vi "trainer on read.vi"(11 "error in (no error)":errorcluster) -> (8 "Trainer is on":bool, 15 "error out":errorcluster)   [LabVIEW 2016]
doc: "this vi reads the trainer 5V power rail using channel 3 to check that the power is on\n\nPaul K Dixon\nPhysics 350\nPaul K Dixon"
panel:
  in  "channel":tag="Dev1/ai3"
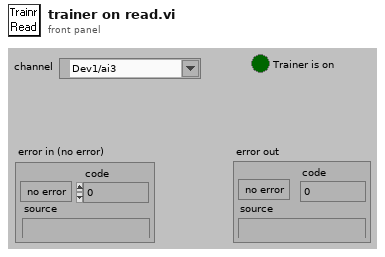
[diagram p1: front panel]
types:
  T1 = enum16{"AI sample channel scan", "AI Waveform triggered"}
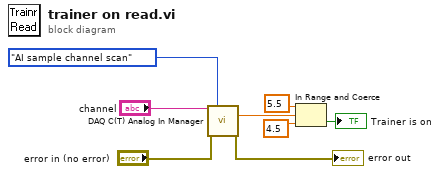
[diagram p0: block diagram]
diagram:
  n1 = call "DAQ C(T) Analog In Manager.vi"("channel (single point) (0)"="channel", "AI mode chooser"=T1."AI sample channel scan", "error in (no error)"="error in (no error)") -> ("V meas"=w3:dbl, "error out"=→"error out":errorcluster)  [unwired: 5 in, 6 out]
  n2 = In Range and Coerce(upper limit=5.5, x=w3, lower limit=4.5) -> (In Range?=→"Trainer is on":bool)  [unwired: 1 out]
